vi "lecturaCluster.vi"() -> ()   [LabVIEW 2011]
panel:
  out "Array":T1(array[cluster]) {"velocidad 3" scale=0.0..180.0; "velocidad 2" scale=0.0..180.0; "velocidad 1" scale=0.0..180.0}
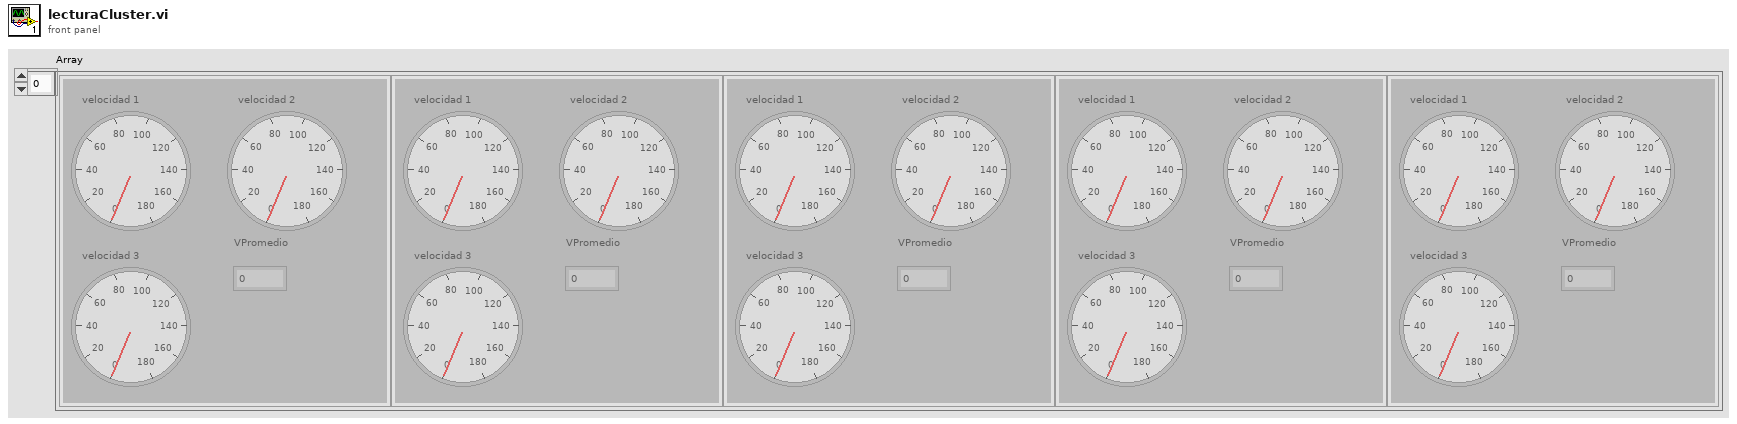
[diagram p1: front panel]
types:
  T1 = cluster{"velocidad 1":i32, "velocidad 2":i32, "velocidad 3":i32, "\n\n\nVPromedio":dbl}[]
  T2 = enum16{"open", "replace", "create", "open or create", "replace or create", "replace or create with confirmation"}
  T3 = cluster{"velocidad 1":i32, "velocidad 2":i32, "velocidad 3":i32, "\n\n\nVPromedio":dbl}
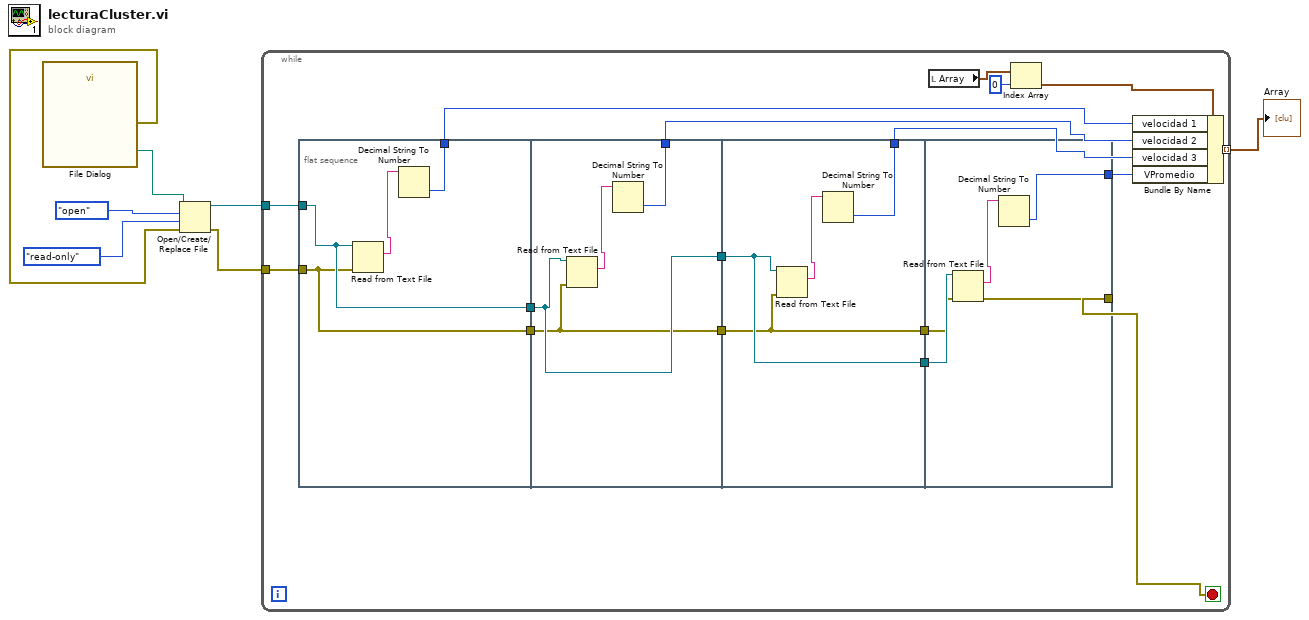
[diagram p0: block diagram]
diagram:
  n1 = call "File Dialog"() -> ("selected path"=w7:path, "error out"=w4:errorcluster)  [unwired: 12 in, 2 out]
  n2 = Open/Create/Replace File(file path (use dialog)=w7, error in=w4, operation (0:open)=T2."open", access (0:read/write)=enum16{"read/write", "read-only", "write-only"}."read-only") -> (refnum out=w3:refnum<file>, error out=w2:errorcluster)  [unwired: 2 in, 1 out]
  n3 = while {
    tunnel: w3 -> [w24]
    tunnel: w2 -> [w23]
    tunnel: [w18] -> w1 mode=indexing
    stop <- w8 stop-if-true
    n4 = flat-sequence {
      tunnel: w24 -> [w26]
      tunnel: w23 -> [w25]
      tunnel: [w27] -> w19
      tunnel: [w26] -> w17
      tunnel: [w25] -> w16
      tunnel: w17 -> [w30]
      tunnel: w16 -> [w29]
      tunnel: [w31] -> w15
      tunnel: [w30] -> w14
      tunnel: [w29] -> w12
      tunnel: w14 -> [w35]
      tunnel: [w35] -> w13
      tunnel: w12 -> [w34]
      tunnel: [w34] -> w11
      tunnel: [w33] -> w10
      tunnel: w13 -> [w40]
      tunnel: w11 -> [w39]
      tunnel: [w38] -> w9
      tunnel: [w37] -> w8
      frame #0 {
        n5 = Read from Text File(file (use dialog)=w26, error in=w25) -> (text=w28:string)  [unwired: 2 in, 3 out]
        n6 = Decimal String To Number(string=w28) -> (number=w27:i32)  [unwired: 2 in, 1 out]
      }
      frame #1 {
        n7 = Read from Text File(file (use dialog)=w30, error in=w29) -> (text=w32:string)  [unwired: 2 in, 3 out]
        n8 = Decimal String To Number(string=w32) -> (number=w31:i32)  [unwired: 2 in, 1 out]
      }
      frame #2 {
        n9 = Read from Text File(file (use dialog)=w35, error in=w34) -> (text=w36:string)  [unwired: 2 in, 3 out]
        n10 = Decimal String To Number(string=w36) -> (number=w33:i32)  [unwired: 2 in, 1 out]
      }
      frame #3 {
        n11 = Read from Text File(file (use dialog)=w40, error in=w39) -> (text=w41:string, error out=w37:errorcluster)  [unwired: 2 in, 2 out]
        n12 = Decimal String To Number(string=w41) -> (number=w38:i32)  [unwired: 2 in, 1 out]
      }
    }
    n13 = local read "Array"() -> (w22:T1)
    n14 = Index Array(array=w22, index=0) -> (element=w20:T3)
    n15 = Bundle By Name "Bundle By Name"(cluster=w20, "velocidad 1"=w19, "velocidad 2"=w15, "velocidad 3"=w10, "VPromedio"=w9) -> (w18:T3)
  }
  "Array" <- w1
